vi "get_visaResource.vi"(0 "HGF_VISADevice":refnum<class "HGF_VISADevice.lvclass">, 5 "error in (no error)":errorcluster) -> (14 "dup HGF_VISADevice":refnum<class "HGF_VISADevice.lvclass">, 16 "VISA Resource Name":refnum<visa-resource-name>, 17 "Serial Configuration":T1, 19 "error out":errorcluster)   [LabVIEW 2014, in "HGF_DeviceBaseClasses.lvlib" / "HGF_VISADevice.lvclass"]
uses:
  HGF_VISADevice.lvclass
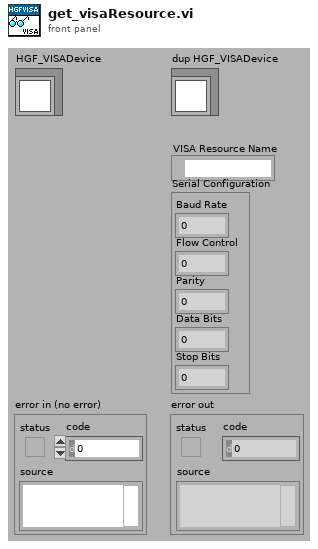
[diagram p1: front panel]
types:
  T1 = cluster{"Baud Rate":u32, "Flow Control":u16, "Parity":u16, "Data Bits":u16, "Stop Bits":u16}
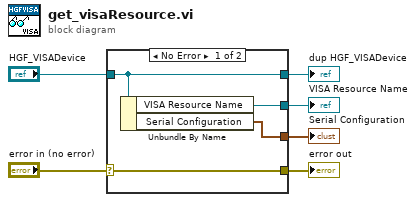
[diagram p0: block diagram]
diagram:
  n1 = case shown="No Error" "error in (no error)" {
    selector: "error in (no error)" -> [w10 w11]
    tunnel: [w10 w11] -> w5
    tunnel: [w9 w12] -> w3
    tunnel: "HGF_VISADevice" -> [w9 w12]
    tunnel: [w8 _] -> w2
    tunnel: [w7 _] -> w1
    frame No Error {
      n2 = Unbundle By Name(w9) -> ("VISA Resource Name"=w8:refnum<visa-resource-name>, "Serial Configuration"=w7:T1)
    }
    frame Error {
    }
  }
  "error out" <- w5
  "dup HGF_VISADevice" <- w3
  "VISA Resource Name" <- w2
  "Serial Configuration" <- w1
